vi "MB Ethernet Example Master.vi"() -> ()   [LabVIEW 2023, in "Voegtlin_NI_SMART_Modbus_Drivers.lvlib"]
uses:
  Voegtlin_NI_SMART_Modbus_Drivers.lvlib
  MB Ethernet Master Query Read Discrete Inputs (poly).vi
  MB Ethernet Master Query Read Input Registers (poly).vi
  MB Ethernet Master Query Write Multiple Registers (poly).vi
  MB Ethernet Master Query Write Multiple Coils (poly).vi
panel:
  in  "Remote IP Address":string="127.0.0.1"
  in  "Remote Port":u16=502
  in  "Stop":bool
  out "Slave Input Registers":u16[](array[numeric]) caption="Slave Input Registers (Read Only)"
  out "Slave Discrete Inputs":bool[](array[boolean])
  in  "Coils to Write":bool[](array[boolean])=[FALSE, FALSE, FALSE, FALSE]
  in  "Registers to Write":u16[](array[numeric])=[0, 0, 0, 0]
  # "MB Ethernet Example Master.vi\n\nInstructions\n1. Run MB Ethernet Example Slave.vi\n2. Run this VI.\n3. Modify the discrete inputs or input registers on the slave -> they're updated on the master.\n4. Modify the coils and registers on the master -> they're updated on the slave."
  # "TCP Parameters"
  # "Data to write to the slave"
  # "Slave Read-only Registers"
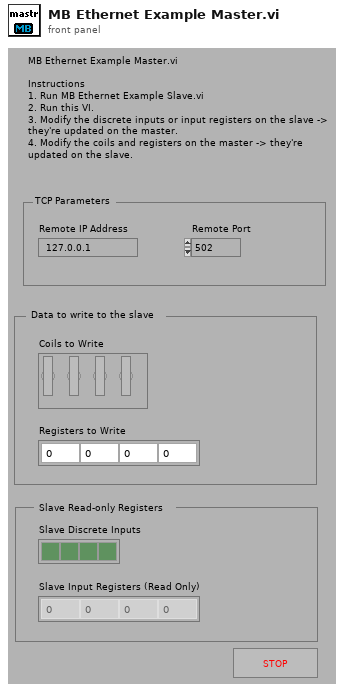
[diagram p1: front panel]
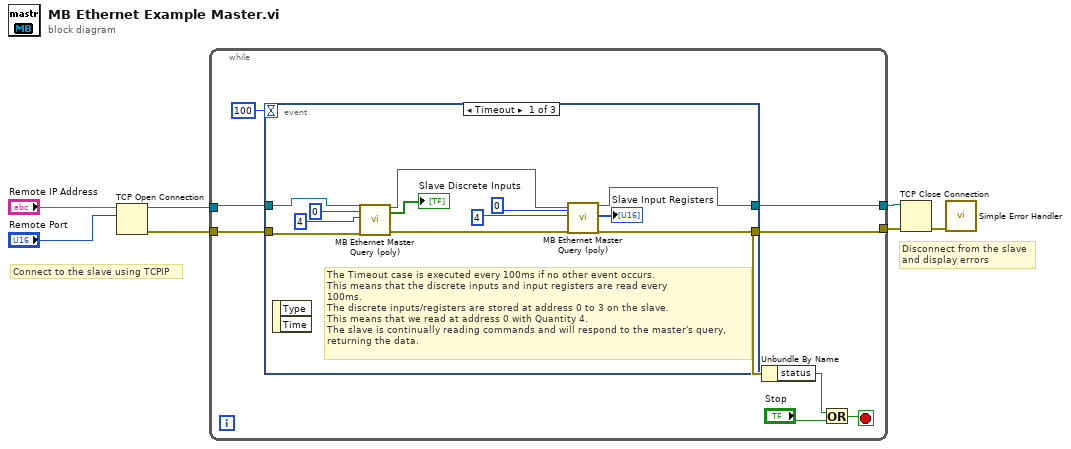
[diagram p0: block diagram]
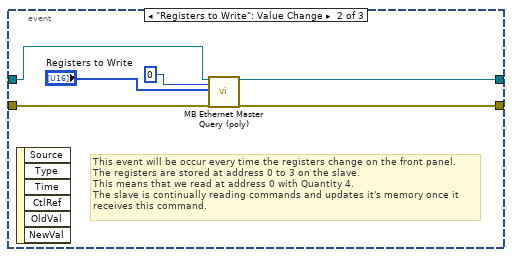
[diagram p2: hidden frame]
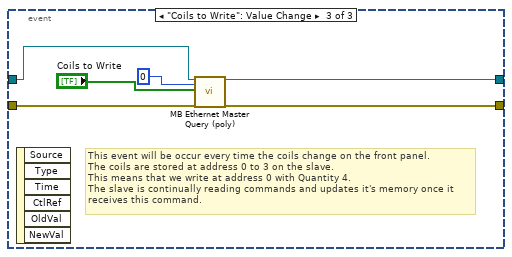
[diagram p3: hidden frame]
diagram:
  # "Disconnect from the slave\nand display errors"
  # "Connect to the slave using TCPIP"
  n1 = TCP Open Connection(address="Remote IP Address", remote port or service name="Remote Port") -> (connection ID=w5:refnum<k5>, error out=w4:errorcluster)  [unwired: 1 in, 2 out]
  n2 = while {
    tunnel: [w12] -> w2
    tunnel: w5 -> [w10]
    tunnel: w4 -> [w9]
    tunnel: [w8] -> w1
    stop <- w15 stop-if-true
    n3 = event shown="[0] Timeout" {
      selector: _ -> [_ _ _]
      dyn-events: _ -> [_ _ _]
      timeout: 100 -> [_ _ _]
      tunnel: [w16 w29 w39] -> w12
      tunnel: w10 -> [w27 w33 w38]
      tunnel: w9 -> [w24 w32 w35]
      tunnel: [w18 w28 w34] -> w8
      event Timeout {
        # "The Timeout case is executed every 100ms if no other event occurs.\nThis means that the discrete inputs and input registers are read every \n100ms.\nThe discrete inputs/registers are stored at address 0 to 3 on the slave.\nThis means that we read at address 0 with Quantity 4.\nThe slave is continually reading commands and will respond to the master's query,\nreturning the data."
        n4 = event-data() -> ()  [unwired: 3 out]
        n5 = call-poly "MB Ethernet Master Query (poly).vi"("TCP Connection Refnum in"=w27, "Starting Address"=u16 0, "Quantity"=u16 4, "error in"=w24) -> ("TCP Connection Refnum (dup)"=w22:refnum<k5>, "Discrete Inputs"=→"Slave Discrete Inputs":bool[], "error out"=w21:errorcluster)  [unwired: 1 in, 12 out]
        n6 = call-poly "MB Ethernet Master Query (poly).vi"("TCP Connection Refnum in"=w22, "Starting Address"=u16 0, "Quantity"=u16 4, "error in"=w21) -> ("TCP Connection Refnum (dup)"=w18:refnum<k5>, "Input Registers"=→"Slave Input Registers":u16[], "error out"=w16:errorcluster)  [unwired: 1 in, 12 out]
      }
      event "Registers to Write": Value Change {
        # "This event will be occur every time the registers change on the front panel.\nThe registers are stored at address 0 to 3 on the slave.\nThis means that we read at address 0 with Quantity 4.\nThe slave is continually reading commands and updates it's memory once it\nreceives this command."
        n7 = event-data() -> ()  [unwired: 7 out]
        n8 = call-poly "MB Ethernet Master Query (poly).vi"("TCP Connection Refnum in"=w33, "Starting Address"=u16 0, "Registers"="Registers to Write", "error in"=w32) -> ("TCP Connection Refnum (dup)"=w28:refnum<k5>, "error out"=w29:errorcluster)  [unwired: 3 in, 11 out]
      }
      event "Coils to Write": Value Change {
        # "This event will be occur every time the coils change on the front panel.\nThe coils are stored at address 0 to 3 on the slave.\nThis means that we write at address 0 with Quantity 4.\nThe slave is continually reading commands and updates it's memory once it\nreceives this command."
        n9 = event-data() -> ()  [unwired: 7 out]
        n10 = call-poly "MB Ethernet Master Query (poly).vi"("TCP Connection Refnum in"=w38, "Starting Address"=u16 0, "Coils"="Coils to Write", "error in"=w35) -> ("TCP Connection Refnum (dup)"=w34:refnum<k5>, "error out"=w39:errorcluster)  [unwired: 3 in, 11 out]
      }
    }
    n11 = Unbundle By Name(w12) -> ("status"=w13:bool)
    n12 = Or(x=w13, y="Stop") -> (x .or. y?=w15:bool)
  }
  n13 = TCP Close Connection(connection ID=w1, error in (no error)=w2) -> (error out=w3:errorcluster)  [unwired: 2 out]
  n14 = call <vilib>:"Simple Error Handler.vi"("error in (no error)"=w3) -> ()  [unwired: 1 in, 8 out]
